vi "InitFileRefs.vi"(8 "error in":errorcluster, 9 "file exists?":bool, 10 "FileRefs":T1 {"Complex"."Group_ref" format="%.0x"; "Complex"."QSpect_dset" format="%.0x"; "Complex"."ISpect_dset" format="%.0x"; "Complex"."PwrSpect_dset" format="%.0x"; "Complex"."TImeStamp_dset" format="%.0x"; "ADAM_Refs"."Group_ref" format="%.0x"; "ADAM_Refs"."ADAM_CoPol_dset" format="%.0x"; "ADAM_Refs"."ADAM_XPol_dset" format="%.0x"; "ADAM_Refs"."ADAM_Noise_dset" format="%.0x"; "ADAM_Refs"."ADAM_CalBox_dset" format="%.0x"; "ADAM_Refs"."TimeStamp" format="%.0x"; "Filter_Refs"."Filter_Group_ref" format="%.0x"; "Filter_Refs"."TimeStamp_dset" format="%.0x"; "Filter_Refs"."Filter_dset" format="%.0x"; "AI_Refs"."BlowerPwr_dset" format="%.0x"; "AI_Refs"."ElStdDev_dset" format="%.0x"; "AI_Refs"."AzStdDev_dset" format="%.0x"; "AI_Refs"."AI19_dset" format="%.0x"; "AI_Refs"."AI18_dset" format="%.0x"; "AI_Refs"."AI17_dset" format="%.0x"; "AI_Refs"."AI16_dset" format="%.0x"; "AI_Refs"."AI6_dset" format="%.0x"; "AI_Refs"."AI5_dset" format="%.0x"; "AI_Refs"."AI4_dset" format="%.0x"; "AI_Refs"."AI3_dset" format="%.0x"; "AI_Refs"."AI2_dset" format="%.0x"; "AI_Refs"."AI0_dset" format="%.0x"; "AI_Refs"."AI1_dset" format="%.0x"; "AI_Refs"."TimeString_dset" format="%.0x"; "AI_Refs"."TimeStamp_dset" format="%.0x"; "AI_Refs"."Group_ref" format="%.0x"; "Weath_Refs"."WindDirSTD_dset" format="%.0x"; "Weath_Refs"."WindGusts_dset" format="%.0x"; "Weath_Refs"."RainFall_dset" format="%.0x"; "Weath_Refs"."RainRate_dset" format="%.0x"; "Weath_Refs"."Pressure_dset" format="%.0x"; "Weath_Refs"."Humidity_dset" format="%.0x"; "Weath_Refs"."Temp_dset" format="%.0x"; "Weath_Refs"."WindDir_dset" format="%.0x"; "Weath_Refs"."WindSpd_dset" format="%.0x"; "Weath_Refs"."TimeStamp_dset" format="%.0x"; "Weath_Refs"."Group_ref" format="%.0x"; "Weath_Refs"."TimeString_dset" format="%.0x"; "UPS_Refs_Deprecated"."TimeStamp_dset" format="%.0x"; "UPS_Refs_Deprecated"."TimeString_dset" format="%.0x"; "UPS_Refs_Deprecated"."%_dset" format="%.0x"; "UPS_Refs_Deprecated"."W_dset" format="%.0x"; "UPS_Refs_Deprecated"."Hz_dset" format="%.0x"; "UPS_Refs_Deprecated"."A_dset" format="%.0x"; "UPS_Refs_Deprecated"."V_dset" format="%.0x"; "UPS_Refs_Deprecated"."Group_ref" format="%.0x"; "TE_Refs"."TimeStamp" format="%.0x"; "TE_Refs"."TE_Outp3_dset" format="%.0x"; "TE_Refs"."TE_Temp3_dset" format="%.0x"; "TE_Refs"."TE_Outp2_dset" format="%.0x"; "TE_Refs"."TE_Temp2_dset" format="%.0x"; "TE_Refs"."TE_Outp1_dset" format="%.0x"; "TE_Refs"."TE_Temp1_dset" format="%.0x"; "TE_Refs"."Group_ref" format="%.0x"; "DisdromRefs"."Status_dset_deprecated" format="%.0x"; "DisdromRefs"."Spectrum_dset" format="%.0x"; "DisdromRefs"."SpectGroup_ref" format="%.0x"; "DisdromRefs"."HydromType_dset" format="%.0x"; "DisdromRefs"."UnknownVolum_dset" format="%.0x"; "DisdromRefs"."UnknownParticls_dset" format="%.0x"; "DisdromRefs"."NonHydrVolum_dset" format="%.0x"; "DisdromRefs"."NonHydrParticls_dset" format="%.0x"; "DisdromRefs"."ParticlMinDiam_dset" format="%.0x"; "DisdromRefs"."ParticlMaxSpeed_dset" format="%.0x"; "DisdromRefs"."RadarReflect_dset" format="%.0x"; "DisdromRefs"."Visibility_dset" format="%.0x"; "DisdromRefs"."TotalRain_dset" format="%.0x"; "DisdromRefs"."Solid_dset" format="%.0x"; "DisdromRefs"."Liquid_dset" format="%.0x"; "DisdromRefs"."TotalRainRate_dset" format="%.0x"; "DisdromRefs"."TimeStamp_dset" format="%.0x"; "DisdromRefs"."ParticlMinSpeed_dset" format="%.0x"; "DisdromRefs"."MeasdParticles_dset" format="%.0x"; "DisdromRefs"."MaxDiam_dset" format="%.0x"; "DisdromRefs"."BasicGroup_ref" format="%.0x"; "ValidRefs"."Alarm_Source_dset" format="%.0x"; "ValidRefs"."Time_AlarmChange_dset" format="%.0x"; "ValidRefs"."Time_Valid_dset" format="%.0x"; "ValidRefs"."Alarm_Valid_dset" format="%.0x"; "ValidRefs"."Saturat_dset" format="%.0x"; "ValidRefs"."Group_ref" format="%.0x"; "ValidRefs"."Weath_Valid_dset" format="%.0x"; "ValidRefs"."Disdr_Valid_dset" format="%.0x"; "TC_Refs"."TC13_Tamb_Inter" format="%.0x"; "TC_Refs"."TC12_Gen_Exhaust" format="%.0x"; "TC_Refs"."TC11_HVAC_Cond_Out" format="%.0x"; "TC_Refs"."TC10_HVAC_Cond_In" format="%.0x"; "TC_Refs"."TC9_LP2_Lo" format="%.0x"; "TC_Refs"."TC8_LP2_LoMid" format="%.0x"; "TC_Refs"."TC7_LP2_Mid" format="%.0x"; "TC_Refs"."TC6_LP2_MidHi" format="%.0x"; "TC_Refs"."TC5_LP2_Hi" format="%.0x"; "TC_Refs"."TC4_LP1_Lo" format="%.0x"; "TC_Refs"."TC3_LP1_LoMid" format="%.0x"; "TC_Refs"."TC2_LP1_Mid" format="%.0x"; "TC_Refs"."TC1_LP1_MidHi" format="%.0x"; "TC_Refs"."TC0_LP1_Hi" format="%.0x"; "TC_Refs"."TimeString_dset" format="%.0x"; "TC_Refs"."TimeStamp_dset" format="%.0x"; "TC_Refs"."Group_ref" format="%.0x"; "NoiseRefs"."TimeStamp_df_dset" format="%.0x"; "NoiseRefs"."sum_dset" format="%.0x"; "NoiseRefs"."df_dset" format="%.0x"; "NoiseRefs"."TimeStamp_dset" format="%.0x"; "NoiseRefs"."SumdSpectrum_dset" format="%.0x"; "NoiseRefs"."TimeString_dset" format="%.0x"; "NoiseRefs"."Group_ref" format="%.0x"; "ToneRefs"."Group_ref" format="%.0x"; "ToneRefs"."Cal"."Downshift_dset" format="%.0x"; "ToneRefs"."Cal"."DeltaPhase_dset" format="%.0x"; "ToneRefs"."Cal"."Phase_dset" format="%.0x"; "ToneRefs"."Cal"."SNR_dset" format="%.0x"; "ToneRefs"."Cal"."df_dset" format="%.0x"; "ToneRefs"."Cal"."PeakLoc_dset" format="%.0x"; "ToneRefs"."Cal"."MaxValue_dset" format="%.0x"; "ToneRefs"."Cal"."TImeStamp_dset" format="%.0x"; "ToneRefs"."Cal"."TimeString_dset" format="%.0x"; "ToneRefs"."Beac"."Downshift_dset" format="%.0x"; "ToneRefs"."Beac"."DeltaPhase_dset" format="%.0x"; "ToneRefs"."Beac"."Phase_dset" format="%.0x"; "ToneRefs"."Beac"."SNR_dset" format="%.0x"; "ToneRefs"."Beac"."df_dset" format="%.0x"; "ToneRefs"."Beac"."PeakLoc_dset" format="%.0x"; "ToneRefs"."Beac"."MaxValue_dset" format="%.0x"; "ToneRefs"."Beac"."TImeStamp_dset" format="%.0x"; "ToneRefs"."Beac"."TimeString_dset" format="%.0x"; "ToneRefs"."CalZoom_dSet" format="%.0x"; "ToneRefs"."BeacZoom_dSet" format="%.0x"; "File" format="%.0x"}, 11 "FileRef":T2 format="%.0x") -> (0 "error out":errorcluster, 2 "FileRefs out":T1 {"Complex"."Group_ref" format="%.0x"; "Complex"."QSpect_dset" format="%.0x"; "Complex"."ISpect_dset" format="%.0x"; "Complex"."PwrSpect_dset" format="%.0x"; "Complex"."TImeStamp_dset" format="%.0x"; "ADAM_Refs"."Group_ref" format="%.0x"; "ADAM_Refs"."ADAM_CoPol_dset" format="%.0x"; "ADAM_Refs"."ADAM_XPol_dset" format="%.0x"; "ADAM_Refs"."ADAM_Noise_dset" format="%.0x"; "ADAM_Refs"."ADAM_CalBox_dset" format="%.0x"; "ADAM_Refs"."TimeStamp" format="%.0x"; "Filter_Refs"."Filter_Group_ref" format="%.0x"; "Filter_Refs"."TimeStamp_dset" format="%.0x"; "Filter_Refs"."Filter_dset" format="%.0x"; "AI_Refs"."BlowerPwr_dset" format="%.0x"; "AI_Refs"."ElStdDev_dset" format="%.0x"; "AI_Refs"."AzStdDev_dset" format="%.0x"; "AI_Refs"."AI19_dset" format="%.0x"; "AI_Refs"."AI18_dset" format="%.0x"; "AI_Refs"."AI17_dset" format="%.0x"; "AI_Refs"."AI16_dset" format="%.0x"; "AI_Refs"."AI6_dset" format="%.0x"; "AI_Refs"."AI5_dset" format="%.0x"; "AI_Refs"."AI4_dset" format="%.0x"; "AI_Refs"."AI3_dset" format="%.0x"; "AI_Refs"."AI2_dset" format="%.0x"; "AI_Refs"."AI0_dset" format="%.0x"; "AI_Refs"."AI1_dset" format="%.0x"; "AI_Refs"."TimeString_dset" format="%.0x"; "AI_Refs"."TimeStamp_dset" format="%.0x"; "AI_Refs"."Group_ref" format="%.0x"; "Weath_Refs"."WindDirSTD_dset" format="%.0x"; "Weath_Refs"."WindGusts_dset" format="%.0x"; "Weath_Refs"."RainFall_dset" format="%.0x"; "Weath_Refs"."RainRate_dset" format="%.0x"; "Weath_Refs"."Pressure_dset" format="%.0x"; "Weath_Refs"."Humidity_dset" format="%.0x"; "Weath_Refs"."Temp_dset" format="%.0x"; "Weath_Refs"."WindDir_dset" format="%.0x"; "Weath_Refs"."WindSpd_dset" format="%.0x"; "Weath_Refs"."TimeStamp_dset" format="%.0x"; "Weath_Refs"."Group_ref" format="%.0x"; "Weath_Refs"."TimeString_dset" format="%.0x"; "UPS_Refs_Deprecated"."TimeStamp_dset" format="%.0x"; "UPS_Refs_Deprecated"."TimeString_dset" format="%.0x"; "UPS_Refs_Deprecated"."%_dset" format="%.0x"; "UPS_Refs_Deprecated"."W_dset" format="%.0x"; "UPS_Refs_Deprecated"."Hz_dset" format="%.0x"; "UPS_Refs_Deprecated"."A_dset" format="%.0x"; "UPS_Refs_Deprecated"."V_dset" format="%.0x"; "UPS_Refs_Deprecated"."Group_ref" format="%.0x"; "TE_Refs"."TimeStamp" format="%.0x"; "TE_Refs"."TE_Outp3_dset" format="%.0x"; "TE_Refs"."TE_Temp3_dset" format="%.0x"; "TE_Refs"."TE_Outp2_dset" format="%.0x"; "TE_Refs"."TE_Temp2_dset" format="%.0x"; "TE_Refs"."TE_Outp1_dset" format="%.0x"; "TE_Refs"."TE_Temp1_dset" format="%.0x"; "TE_Refs"."Group_ref" format="%.0x"; "DisdromRefs"."Status_dset_deprecated" format="%.0x"; "DisdromRefs"."Spectrum_dset" format="%.0x"; "DisdromRefs"."SpectGroup_ref" format="%.0x"; "DisdromRefs"."HydromType_dset" format="%.0x"; "DisdromRefs"."UnknownVolum_dset" format="%.0x"; "DisdromRefs"."UnknownParticls_dset" format="%.0x"; "DisdromRefs"."NonHydrVolum_dset" format="%.0x"; "DisdromRefs"."NonHydrParticls_dset" format="%.0x"; "DisdromRefs"."ParticlMinDiam_dset" format="%.0x"; "DisdromRefs"."ParticlMaxSpeed_dset" format="%.0x"; "DisdromRefs"."RadarReflect_dset" format="%.0x"; "DisdromRefs"."Visibility_dset" format="%.0x"; "DisdromRefs"."TotalRain_dset" format="%.0x"; "DisdromRefs"."Solid_dset" format="%.0x"; "DisdromRefs"."Liquid_dset" format="%.0x"; "DisdromRefs"."TotalRainRate_dset" format="%.0x"; "DisdromRefs"."TimeStamp_dset" format="%.0x"; "DisdromRefs"."ParticlMinSpeed_dset" format="%.0x"; "DisdromRefs"."MeasdParticles_dset" format="%.0x"; "DisdromRefs"."MaxDiam_dset" format="%.0x"; "DisdromRefs"."BasicGroup_ref" format="%.0x"; "ValidRefs"."Alarm_Source_dset" format="%.0x"; "ValidRefs"."Time_AlarmChange_dset" format="%.0x"; "ValidRefs"."Time_Valid_dset" format="%.0x"; "ValidRefs"."Alarm_Valid_dset" format="%.0x"; "ValidRefs"."Saturat_dset" format="%.0x"; "ValidRefs"."Group_ref" format="%.0x"; "ValidRefs"."Weath_Valid_dset" format="%.0x"; "ValidRefs"."Disdr_Valid_dset" format="%.0x"; "TC_Refs"."TC13_Tamb_Inter" format="%.0x"; "TC_Refs"."TC12_Gen_Exhaust" format="%.0x"; "TC_Refs"."TC11_HVAC_Cond_Out" format="%.0x"; "TC_Refs"."TC10_HVAC_Cond_In" format="%.0x"; "TC_Refs"."TC9_LP2_Lo" format="%.0x"; "TC_Refs"."TC8_LP2_LoMid" format="%.0x"; "TC_Refs"."TC7_LP2_Mid" format="%.0x"; "TC_Refs"."TC6_LP2_MidHi" format="%.0x"; "TC_Refs"."TC5_LP2_Hi" format="%.0x"; "TC_Refs"."TC4_LP1_Lo" format="%.0x"; "TC_Refs"."TC3_LP1_LoMid" format="%.0x"; "TC_Refs"."TC2_LP1_Mid" format="%.0x"; "TC_Refs"."TC1_LP1_MidHi" format="%.0x"; "TC_Refs"."TC0_LP1_Hi" format="%.0x"; "TC_Refs"."TimeString_dset" format="%.0x"; "TC_Refs"."TimeStamp_dset" format="%.0x"; "TC_Refs"."Group_ref" format="%.0x"; "NoiseRefs"."TimeStamp_df_dset" format="%.0x"; "NoiseRefs"."sum_dset" format="%.0x"; "NoiseRefs"."df_dset" format="%.0x"; "NoiseRefs"."TimeStamp_dset" format="%.0x"; "NoiseRefs"."SumdSpectrum_dset" format="%.0x"; "NoiseRefs"."TimeString_dset" format="%.0x"; "NoiseRefs"."Group_ref" format="%.0x"; "ToneRefs"."Group_ref" format="%.0x"; "ToneRefs"."Cal"."Downshift_dset" format="%.0x"; "ToneRefs"."Cal"."DeltaPhase_dset" format="%.0x"; "ToneRefs"."Cal"."Phase_dset" format="%.0x"; "ToneRefs"."Cal"."SNR_dset" format="%.0x"; "ToneRefs"."Cal"."df_dset" format="%.0x"; "ToneRefs"."Cal"."PeakLoc_dset" format="%.0x"; "ToneRefs"."Cal"."MaxValue_dset" format="%.0x"; "ToneRefs"."Cal"."TImeStamp_dset" format="%.0x"; "ToneRefs"."Cal"."TimeString_dset" format="%.0x"; "ToneRefs"."Beac"."Downshift_dset" format="%.0x"; "ToneRefs"."Beac"."DeltaPhase_dset" format="%.0x"; "ToneRefs"."Beac"."Phase_dset" format="%.0x"; "ToneRefs"."Beac"."SNR_dset" format="%.0x"; "ToneRefs"."Beac"."df_dset" format="%.0x"; "ToneRefs"."Beac"."PeakLoc_dset" format="%.0x"; "ToneRefs"."Beac"."MaxValue_dset" format="%.0x"; "ToneRefs"."Beac"."TImeStamp_dset" format="%.0x"; "ToneRefs"."Beac"."TimeString_dset" format="%.0x"; "ToneRefs"."CalZoom_dSet" format="%.0x"; "ToneRefs"."BeacZoom_dSet" format="%.0x"; "File" format="%.0x"})   [LabVIEW 2018]
uses:
  <vilib>/addons/h5labview2/base/hid_t.ctl
  Controls/Clusts/HDF5_File_Refs.ctl
  Controls/Clusts/ToneGroupRefsClust.ctl
  HDF5/HDF5_Tone_refs.ctl
  HDF5/HDF5_Noise_refs.ctl
  HDF5/TC_Tone_refs.ctl
  HDF5/HDF5_Validty_refs.ctl
  HDF5/HDF5_Disdrometer_Refs.ctl
  HDF5/HDF5_Health_Refs.ctl
  HDF5/UPS_refs.ctl
  Controls/Clusts/WeatherRefs.ctl
  HDF5/HDF5_AI_refs.ctl
  HDF5/HDF5_Filter_refs.ctl
  HDF5/HDF5_ADAM_Refs.ctl
  HDF5/HDF5_Complex_Refs.ctl
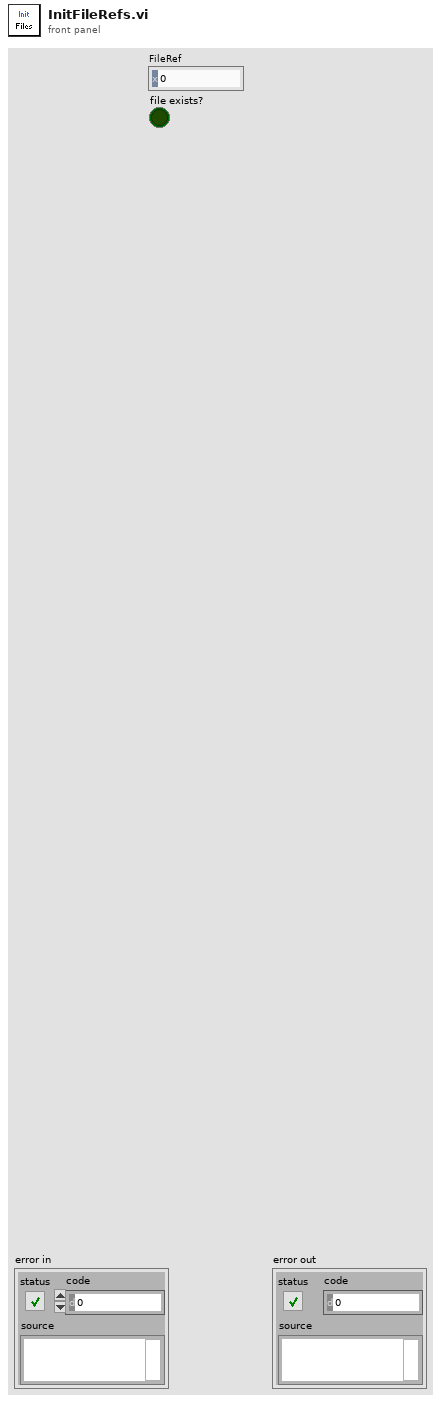
[diagram p1: front panel]
types:
  T1 = typedef "HDF5_File_Refs.ctl" = cluster{"File":T2, "ToneRefs":T3[], "NoiseRefs":T5[], "TC_Refs":T6, "ValidRefs":T7, "DisdromRefs":T8, "TE_Refs":T9, "UPS_Refs_Deprecated":T10, "Weath_Refs":T11, "AI_Refs":T12, "Filter_Refs":T13, "ADAM_Refs":T14, "Complex":T15[]}
  T2 = typedef "hid_t.ctl" = i32
  T3 = typedef "ToneGroupRefsClust.ctl" = cluster{"Group_ref":T2, "Cal":T4, "Beac":T4, "CalZoom_dSet":T2, "BeacZoom_dSet":T2}
  T4 = typedef "HDF5_Tone_refs.ctl" = cluster{"TimeString_dset":T2, "TImeStamp_dset":T2, "SNR_dset":T2, "MaxValue_dset":T2, "PeakLoc_dset":T2, "df_dset":T2, "Phase_dset":T2, "DeltaPhase_dset":T2, "Downshift_dset":T2}
  T5 = typedef "HDF5_Noise_refs.ctl" = cluster{"Group_ref":T2, "TimeString_dset":T2, "TimeStamp_dset":T2, "TimeStamp_df_dset":T2, "df_dset":T2, "sum_dset":T2, "SumdSpectrum_dset":T2}
  T6 = typedef "TC_Tone_refs.ctl" = cluster{"Group_ref":T2, "TimeString_dset":T2, "TimeStamp_dset":T2, "TC0_LP1_Hi":T2, "TC1_LP1_MidHi":T2, "TC2_LP1_Mid":T2, "TC3_LP1_LoMid":T2, "TC4_LP1_Lo":T2, "TC5_LP2_Hi":T2, "TC6_LP2_MidHi":T2, "TC7_LP2_Mid":T2, "TC8_LP2_LoMid":T2, "TC9_LP2_Lo":T2, "TC10_HVAC_Cond_In":T2, "TC11_HVAC_Cond_Out":T2, "TC12_Gen_Exhaust":T2, "TC13_Tamb_Inter":T2}
  T7 = typedef "HDF5_Validty_refs.ctl" = cluster{"Group_ref":T2, "Weath_Valid_dset":T2, "Disdr_Valid_dset":T2, "Saturat_dset":T2, "Alarm_Valid_dset":T2, "Time_Valid_dset":T2, "Time_AlarmChange_dset":T2, "Alarm_Source_dset":T2}
  T8 = typedef "HDF5_Disdrometer_Refs.ctl" = cluster{"BasicGroup_ref":T2, "TimeStamp_dset":T2, "TotalRainRate_dset":T2, "Liquid_dset":T2, "Solid_dset":T2, "TotalRain_dset":T2, "Visibility_dset":T2, "RadarReflect_dset":T2, "MaxDiam_dset":T2, "MeasdParticles_dset":T2, "ParticlMinSpeed_dset":T2, "ParticlMaxSpeed_dset":T2, "ParticlMinDiam_dset":T2, "NonHydrParticls_dset":T2, "NonHydrVolum_dset":T2, "UnknownParticls_dset":T2, "UnknownVolum_dset":T2, "HydromType_dset":T2, "SpectGroup_ref":T2, "Spectrum_dset":T2, "Status_dset_deprecated":T2}
  T9 = typedef "HDF5_Health_Refs.ctl" = cluster{"Group_ref":T2, "TE_Temp1_dset":T2, "TE_Outp1_dset":T2, "TE_Temp2_dset":T2, "TE_Outp2_dset":T2, "TE_Temp3_dset":T2, "TE_Outp3_dset":T2, "TimeStamp":T2}
  T10 = typedef "UPS_refs.ctl" = cluster{"Group_ref":T2, "TimeString_dset":T2, "TimeStamp_dset":T2, "V_dset":T2, "A_dset":T2, "Hz_dset":T2, "W_dset":T2, "%_dset":T2}
  T11 = typedef "WeatherRefs.ctl" = cluster{"Group_ref":T2, "TimeString_dset":T2, "TimeStamp_dset ":T2, "WindSpd_dset":T2, "WindGusts_dset":T2, "WindDir_dset":T2, "WindDirSTD_dset":T2, "Temp_dset":T2, "Humidity_dset":T2, "Pressure_dset":T2, "RainRate_dset":T2, "RainFall_dset":T2}
  T12 = typedef "HDF5_AI_refs.ctl" = cluster{"Group_ref":T2, "TimeString_dset":T2, "TimeStamp_dset":T2, "AI0_dset":T2, "AI1_dset":T2, "AI2_dset":T2, "AI3_dset":T2, "AI4_dset":T2, "AI5_dset":T2, "AI6_dset":T2, "AI16_dset":T2, "AI17_dset":T2, "AI18_dset":T2, "AzStdDev_dset":T2, "AI19_dset":T2, "ElStdDev_dset":T2, "BlowerPwr_dset":T2}
  T13 = typedef "HDF5_Filter_refs.ctl" = cluster{"Filter_Group_ref":T2, "TimeStamp_dset":T2, "Filter_dset":T2}
  T14 = typedef "HDF5_ADAM_Refs.ctl" = cluster{"Group_ref":T2, "ADAM_CoPol_dset":T2, "ADAM_XPol_dset":T2, "ADAM_Noise_dset":T2, "ADAM_CalBox_dset":T2, "TimeStamp":T2}
  T15 = typedef "HDF5_Complex_Refs.ctl" = cluster{"Group_ref":T2, "TImeStamp_dset":T2, "PwrSpect_dset":T2, "ISpect_dset":T2, "QSpect_dset":T2}
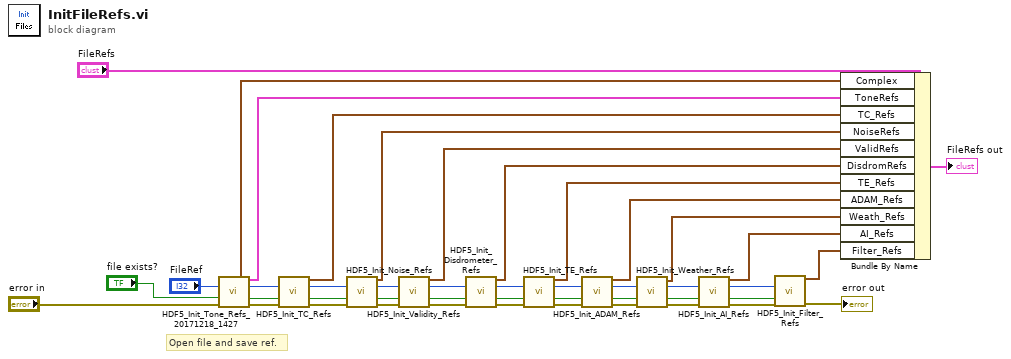
[diagram p0: block diagram]
diagram:
  # "Open file and save ref."
  n1 = call "HDF5_Init_Tone_Refs_20171218_1427.vi"("HDF5 file ref"="FileRef", "File Exists?"="file exists?", "error in"="error in") -> ("ComplexRefs"=w5:T15[], "ToneRefs"=w22:T3[], "HDF5 file ref"=w24:T2, "error out"=w23:errorcluster)  [unwired: 9 in]
  n2 = call "HDF5_Init_TC_Refs.vi"("HDF5 file ref"=w24, "File Exists?"="file exists?", "error in"=w23) -> ("TC_Refs"=w26:T6, "HDF5 file ref"=w27:T2, "error out"=w25:errorcluster)  [unwired: 10 in]
  n3 = call "HDF5_Init_Noise_Refs.vi"("HDF5 file ref"=w27, "File Exists?"="file exists?", "error in"=w25) -> ("NoiseRefs"=w28:T5[], "HDF5 file ref"=w9:T2, "error out"=w29:errorcluster)  [unwired: 10 in]
  n4 = call "HDF5_Init_Validity_Refs.vi"("HDF5 file ref"=w9, "File Exists?"="file exists?", "error in"=w29) -> ("AlarmFileRefs"=w30:T7, "error out"=w20:errorcluster)  [unwired: 11 in]
  n5 = call "HDF5_Init_Disdrometer_Refs.vi"("HDF5 file ref"=w9, "File Exists?"="file exists?", "error in"=w20) -> ("DisdromRefs"=w6:T8, "error out"=w19:errorcluster)  [unwired: 11 in]
  n6 = call "HDF5_Init_TE_Refs.vi"("HDF5 file ref"=w9, "File Exists?"="file exists?", "error in"=w19) -> ("Health_Refs"=w7:T9, "error out"=w11:errorcluster)  [unwired: 11 in]
  n7 = call "HDF5_Init_ADAM_Refs.vi"("HDF5 file ref"=w9, "File Exists?"="file exists?", "error in"=w11) -> ("Health_Refs"=w8:T14, "error out"=w10:errorcluster)  [unwired: 11 in]
  n8 = call "HDF5_Init_Weather_Refs.vi"("error in"=w10, "File Exists?"="file exists?", "HDF5 file ref 2"=w9) -> ("error out"=w17:errorcluster, "HDF5 file ref"=w12:T2, "Weath_Refs"=w18:T11)  [unwired: 6 in]
  n9 = call "HDF5_Init_AI_Refs.vi"("HDF5 file ref"=w12, "File Exists?"="file exists?", "error in"=w17) -> ("AI_Refs"=w16:T12, "error out"=w15:errorcluster)  [unwired: 11 in]
  n10 = call "HDF5_Init_Filter_Refs.vi"("HDF5 file ref"=w12, "File Exists?"="file exists?", "error in"=w15) -> ("Filter_Refs"=w13:T13, "error out"=→"error out":errorcluster)  [unwired: 10 in, 1 out]
  n11 = Bundle By Name(cluster="FileRefs", "Complex"=w5, "ToneRefs"=w22, "TC_Refs"=w26, "NoiseRefs"=w28, "ValidRefs"=w30, "DisdromRefs"=w6, "TE_Refs"=w7, "ADAM_Refs"=w8, "Weath_Refs"=w18, "AI_Refs"=w16, "Filter_Refs"=w13) -> (→"FileRefs out":T1)
